vi "Render.vi"(8 "error in (no error)":errorcluster, 11 "Bouncer in":refnum<class "Bouncer.lvclass">) -> (0 "error out":errorcluster, 3 "Bouncer out":refnum<class "Bouncer.lvclass">)   [LabVIEW 2019, in "RT_Game.lvlib" / "Bouncer.lvclass"]
uses:
  Bouncer.lvclass
  Game/Game.lvclass
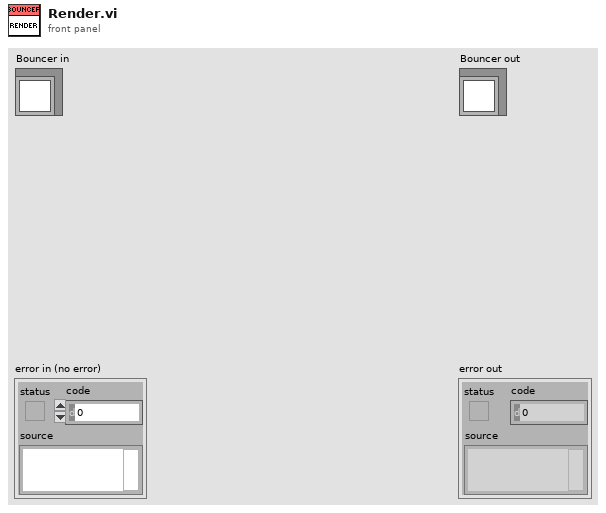
[diagram p1: front panel]
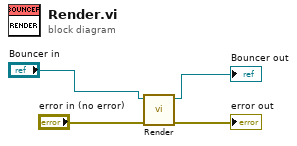
[diagram p0: block diagram]
diagram:
  n1 = call-parent "Render.vi"("error in (no error)"="error in (no error)", "Game in"="Bouncer in") -> ("error out"=→"error out":errorcluster, "Game out"=→"Bouncer out":refnum<class "Bouncer.lvclass">)  [unwired: 8 in]
